vi "Write StringFileGcode.vi"(8 "error in (no error)":errorcluster, 10 "StringFileGcode":string, 11 "ParameterConf in":refnum<class "ParameterConf.lvclass">) -> (0 "error out":errorcluster, 3 "ParameterConf out":refnum<class "ParameterConf.lvclass">)   [LabVIEW 2017, in "ParameterConf.lvclass"]
uses:
  ParameterConf.lvclass
  ParameterConf.lvclass/ParameterConf.ctl
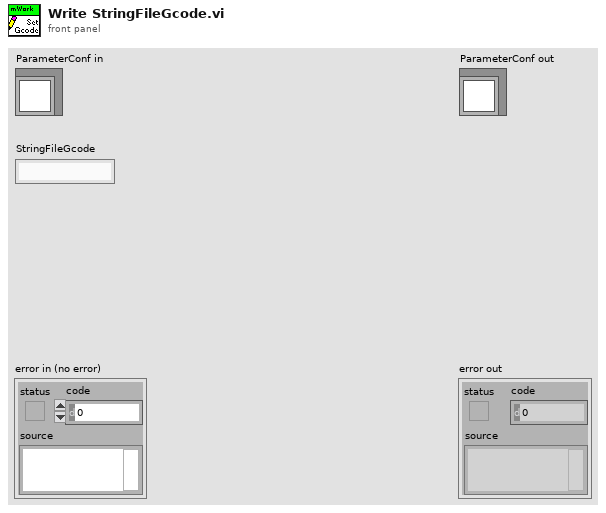
[diagram p1: front panel]
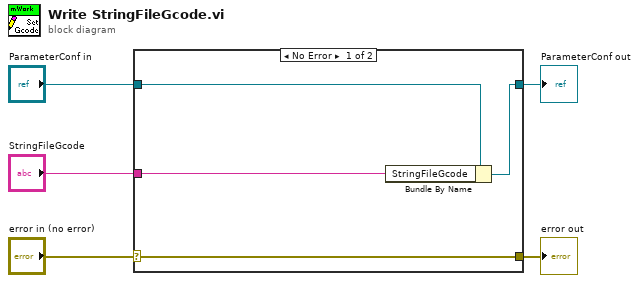
[diagram p0: block diagram]
diagram:
  n1 = case shown="No Error" "error in (no error)" {
    selector: "error in (no error)" -> [w9 w10]
    tunnel: [w9 w10] -> w4
    tunnel: [w7 w11] -> w2
    tunnel: "ParameterConf in" -> [w8 w11]
    tunnel: "StringFileGcode" -> [w6 _]
    frame No Error {
      n2 = Bundle By Name(cluster=w8, "StringFileGcode"=w6) -> (w7:refnum<class "ParameterConf.lvclass">)
    }
    frame Error {
    }
  }
  "error out" <- w4
  "ParameterConf out" <- w2
